vi "Configure Sample Clock Output Enabled [SC] Core.vi"(8 "error in (no error)":errorcluster, 9 "Sample Clock Output Enabled (Disabled)":bool caption="sample clock output enabled (Disabled)", 11 "IVI_Fgen in":refnum<class "IVI_Fgen.lvclass">) -> (0 "error out":errorcluster, 3 "IVI_Fgen out":refnum<class "IVI_Fgen.lvclass">)   [LabVIEW 2015, in "IVI_Fgen.lvlib" / "IVI_Fgen.lvclass"]
doc: "This VI configures whether the sample clock appears at the sample clock output of the generator.\n\nNote:\n\n(1) This VI is part of the IviFgenSampleClock [SC] extension group."
uses:
  IVI_Fgen.lvclass
  IVI_Fgen.lvclass/IVI_Fgen.ctl
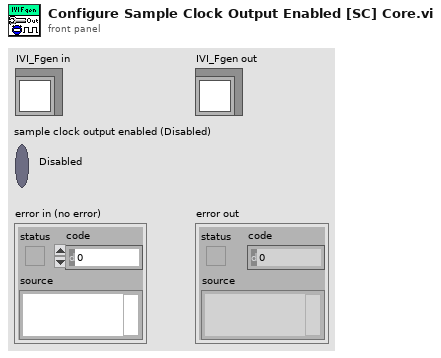
[diagram p1: front panel]
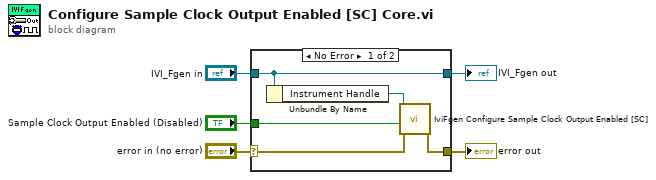
[diagram p0: block diagram]
diagram:
  n1 = case shown="No Error" "error in (no error)" {
    selector: "error in (no error)" -> [w8 w12]
    tunnel: [w7 w12] -> w4
    tunnel: [w10 w11] -> w2
    tunnel: "IVI_Fgen in" -> [w10 w11]
    tunnel: "Sample Clock Output Enabled (Disabled)" -> [w6 _]
    frame No Error {
      n2 = Unbundle By Name(w10) -> ("Instrument Handle"=w9:refnum<k15>)
      n3 = call <vilib>:"IviFgen Configure Sample Clock Output Enabled [SC].vi"("error in (no error)"=w8, "Sample Clock Output Enabled (Disabled)"=w6, "instrument handle"=w9) -> ("error out"=w7:errorcluster)  [unwired: 7 in, 1 out]
    }
    frame Error {
    }
  }
  "error out" <- w4
  "IVI_Fgen out" <- w2
